vi "Read JSON Config.vi"(8 "error in (no error)":errorcluster, 10 "JSON Config":string, 11 "AbsComp_One Term_I16 in":refnum<class "AbsComp_One Term_I16.lvclass">) -> (0 "error out":errorcluster, 3 "AbsComp_One Term_I16 out":refnum<class "AbsComp_One Term_I16.lvclass">)   [LabVIEW 2021, in "AbsComp_One Term_I16.lvclass"]
uses:
  AbsComp_One Term_I16.lvclass
  C:/Program Files (x86)/National Instruments/LabVIEW 2021/vi.lib/TSA/Abstract Data Classes/Abs_Types/Type/Abs_Type.lvclass
  AbsComp_One Term_I16.lvclass/AbsComp_One Term_I16.ctl
  Abs_Types/I16 Integer/Abs_I16 Integer.lvclass
  <vilib>/Utility/LVClass/Get LV Class Name.vi
  Abs_Types/Boolean/Abs_Boolean.lvclass
  Abs_Types/Type/Abs_Type.lvclass
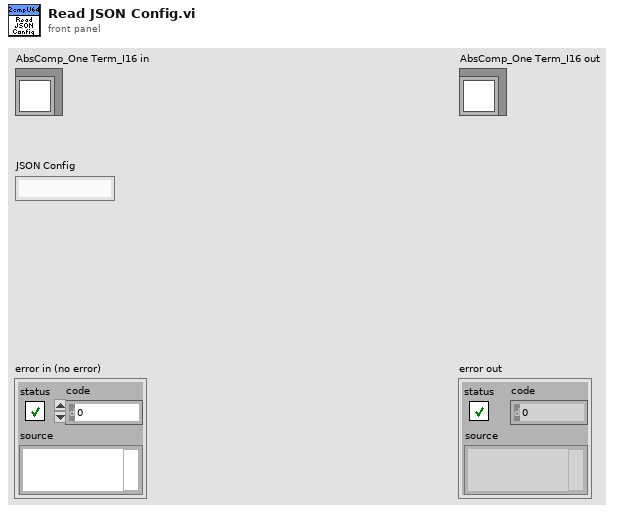
[diagram p1: front panel]
types:
  T1 = typedef "AbsComp_One Term_I16.lvclass/Abstract Type.ctl" = refnum<class "Abs_I16 Integer.lvclass">
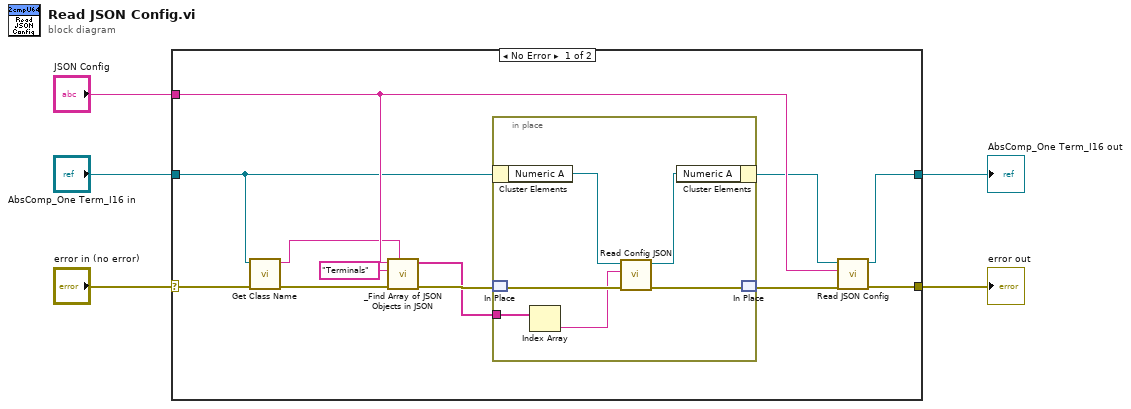
[diagram p0: block diagram]
diagram:
  n1 = case shown="No Error" "error in (no error)" {
    selector: "error in (no error)" -> [w13 w24]
    tunnel: [w17 w24] -> w3
    tunnel: [w16 w25] -> w2
    tunnel: "JSON Config" -> [w15 _]
    tunnel: "AbsComp_One Term_I16 in" -> [w12 w25]
    frame No Error {
      n2 = call "Get Class Name.vi"("error in (no error)"=w13, "Abs_Type in"=w12) -> ("error out"=w14:errorcluster, "class name"=w7:string)  [unwired: 8 in]
      n3 = call "_Find Array of JSON Objects in JSON.vi"("JSON Object Name"=w7, "error in (no error)"=w14, "JSON Array Name"="Terminals", "JSON Config"=w15) -> ("error out"=w11:errorcluster, "JSON Objects"=w10:string[])  [unwired: 6 in]
      n4 = in-place {
        in-place-border: w10 -> [w23]
        n5 = in-place-cluster #1(w12) -> ("Numeric A"=w19:T1)
        n6 = in-place-match #2(w11) -> (w22:errorcluster)
        n7 = Index Array(array=w23) -> (element=w21:string)  [unwired: 1 in]
        n8 = call "Read Config JSON.vi"("error in (no error)"=w22, "JSON Config"=w21, "Abs_Type in"=w19) -> ("error out"=w20:errorcluster, "Abs_Type out"=w18:T1)  [unwired: 7 in]
        n9 = in-place-cluster #1("Numeric A"=w18) -> (w8:refnum<class "AbsComp_One Term_I16.lvclass">)
        n10 = in-place-match #2(w20) -> (w9:errorcluster)
      }
      n11 = call-parent "Read JSON Config.vi"("error in (no error)"=w9, "JSON Config"=w15, "Abs_Type in"=w8) -> ("error out"=w17:errorcluster, "Abs_Type out"=w16:refnum<class "AbsComp_One Term_I16.lvclass">)  [unwired: 7 in]
    }
    frame Error {
    }
  }
  "error out" <- w3
  "AbsComp_One Term_I16 out" <- w2
